vi "phasemeasurement_sine_singletone.vi"() -> ()   [LabVIEW 2018]
uses:
  <vilib>/measure/matone.llb/Extract Single Tone Information 1 Chan.vi
  <vilib>/measure/NI_MAPro.lvlib
panel:
  out "Waveform Graph":waveform(dbl)[](graph)
  out "detected amplitude":dbl format="%.2p"
  out "detected frequency":dbl format="%.2p"
  out "Phase difference (deg)":dbl
  in  "Noise Standard deviation":dbl=0.1 caption="Standard deviation"
  in  "Frequnecy":dbl(knob)=100.0 scale=90.0..110.0
  in  "Phase diference (deg)":dbl=180.0 format="%#_13g"
  # "Signal 2 (inputs)"
  # "Results (output)"
  # "Note:\n1) If you set the stadard deviation to 0 (volt) you get a perfect measurement\n2) Even with high noise, e.g. 0.5 V, you get realtive good mesurements due\n    to the use of an FFT method.\n3) Adding a filter (on both channels to avoid additional phase) does not \n    improve the results significatnly due to the use of an FFT-based method\n4) You cal also change the type of signals, e.g. into Triangle\n5) In this example the sample rate is 20 kHz. If it was lowered to for instace \n    1k Hz (10 times higer than the signal) the result would be less accurate.\n6) The method also work when the frequency is not identica, e.g set Signal 2\n    to have a frequency of 106 Hz"
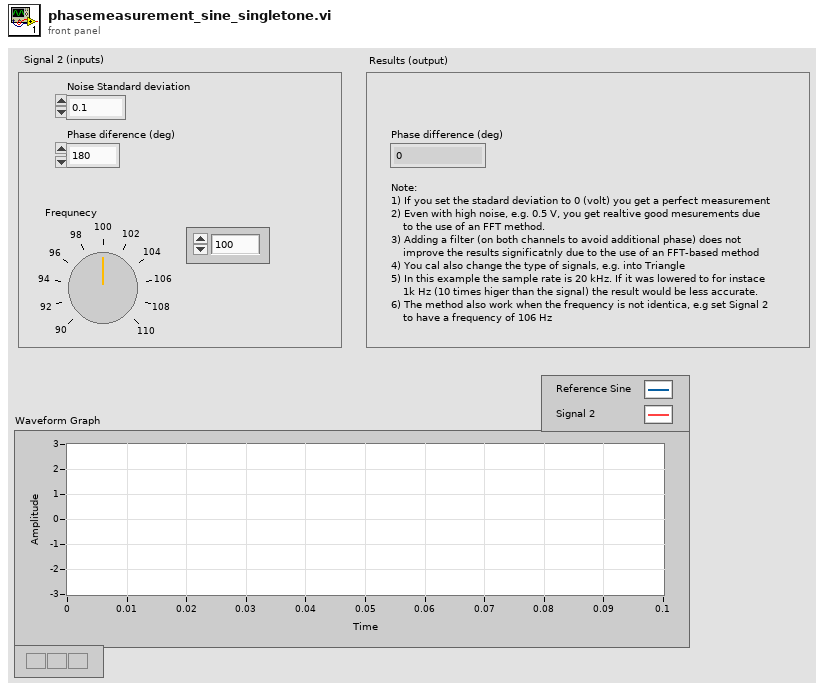
[diagram p1: front panel]
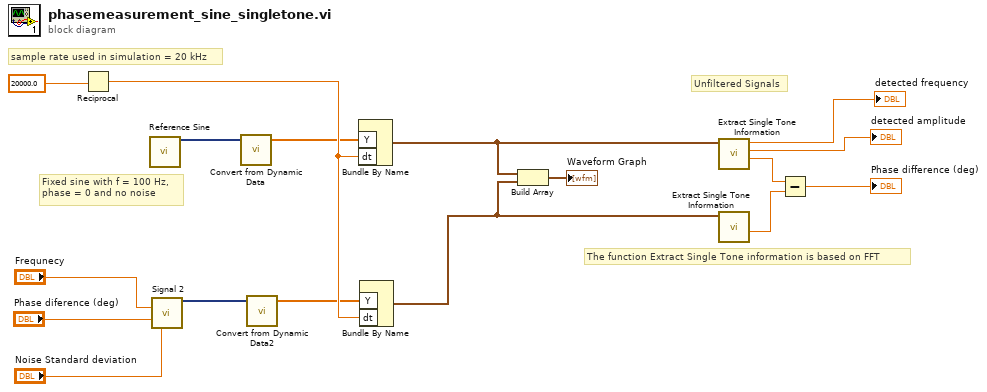
[diagram p0: block diagram]
diagram:
  # "The function Extract Single Tone information is based on FFT"
  # "Unfiltered Signals"
  # "sample rate used in simulation = 20 kHz"
  # "Fixed sine with f = 100 Hz, \nphase = 0 and no noise"
  n1 = Reciprocal(x=20000.0) -> (1/x=w13:dbl)
  n2 = call "Reference Sine"() -> ("Sine100ph0"=w4:dynamicdata)  [unwired: 14 in, 1 out]
  n3 = call "Signal 2"("Frequency"="Frequnecy", "Phase"="Phase diference (deg)", "Standard deviation"="Noise Standard deviation") -> ("SignalVar"=w3:dynamicdata)  [unwired: 11 in, 1 out]
  n4 = call "Convert from Dynamic Data"("Dynamic Data Type"=w4) -> ("Array"=w2:dbl[])  [unwired: 3 in]
  n5 = call "Convert from Dynamic Data2"("Dynamic Data Type"=w3) -> ("Array"=w1:dbl[])  [unwired: 3 in]
  n6 = Bundle By Name("Y"=w2, "dt"=w13) -> (w7:waveform(dbl))  [unwired: 1 in]
  n7 = Bundle By Name("Y"=w1, "dt"=w13) -> (w6:waveform(dbl))  [unwired: 1 in]
  n8 = Build Array(w7, w6) -> (→"Waveform Graph":waveform(dbl)[])
  n9 = call-poly <vilib>:"Extract Single Tone Information.vi"("time signal in"=w7) -> ("detected phase (deg)"=w10:dbl, "detected amplitude"=→"detected amplitude":dbl, "detected frequency"=→"detected frequency":dbl)  [unwired: 5 in, 3 out]
  n10 = call-poly <vilib>:"Extract Single Tone Information.vi"("time signal in"=w6) -> ("detected phase (deg)"=w9:dbl)  [unwired: 5 in, 5 out]
  n11 = Subtract(x=w10, y=w9) -> (x-y=→"Phase difference (deg)":dbl)
